vi "Save and Load Filter to and from Text File.vi"() -> ()   [LabVIEW 2023]
doc: "Demonstrates how to use the DFD Save to Text File VI to save a filter as a text file. This VI also demonstrates how to use the DFD Load from Text File VI to load a filter from a text file. \n\nComplete the following steps to use this VI.\n1) Run the VI.\n2) On the dialog box that appears, specify the path to the file in which you want to save the filter and click the <B>OK</B> button.\n3) Observe the Magnitude Responses graph. The Original Filter plot shows the magnitude response of the original filter. The Filter from File plot shows the magnitude response of the filter that the VI loads from the text file that you specified in Step 2.\n4) Examine the block diagram to learn how to use the Utilities VIs."
uses:
  <vilib>/addons/Digital Filter Design/_Objects.llb/DFD Filter Ripple Specification (Design).ctl
  <vilib>/addons/Digital Filter Design/_Objects.llb/DFD Filter Frequence Specification (Design).ctl
  <vilib>/addons/Digital Filter Design/Analysis.llb/DFD Plot Freq Response (Linear-Spaced).vi
  <vilib>/addons/Digital Filter Design/FilterLib.llb/DFD Save Filter to Text File.vi
  <vilib>/addons/Digital Filter Design/FilterLib.llb/DFD Load Filter from Text File.vi
  <vilib>/addons/Digital Filter Design/NI_DigFilterLicensed.lvlib
panel:
  out "Text":string
  in  "Load Type":u16(ring) items=["From Coefficients", "From Zero-Pole-Gain"]
  in  "Design Method":T1(ring)=enum."Elliptic"
  out "Magnitude Responses":cluster{"f0":dbl, "df":dbl, "values":dbl[]}[](graph)
  in  "Filter Type":u16(ring) items=["Lowpass", "Highpass", "Bandpass", "Bandstop"]
  in  "Frequency Sepcifications [Hz]":T2={"fpass 1"=100.0, "fstop 1"=200.0, "fpass 2 "=0.0, "fstop 2"=0.0}
  in  "Ripple Specifications":T3={"passband"=0.1, "stopband"=60.0, "dB/linear? (T: dB)"=TRUE}
  in  "Sampling Frequency [Hz]":dbl=1000.0 format="%.2f"
  out "Error Message":string
  # "Select Help>>Show Context Help and move the cursor over the VI icon for more information."
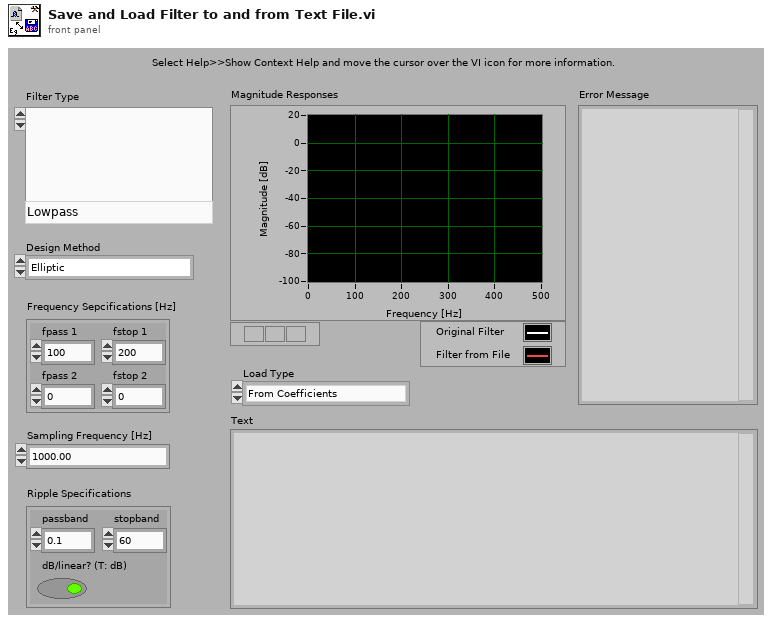
[diagram p1: front panel]
types:
  T1 = enum16{"Butterworth", "Chebyshev", "Inverse Chebyshev", "Elliptic", "Kaiser Window", "Dolph-Chebyshev Window", "Equi-Ripple FIR"}
  T2 = typedef "NI_DigFilterLicensed.lvlib/DFD Filter Frequence Specification (Design).ctl" = cluster{"fpass 1":dbl, "fstop 1":dbl, "fpass 2 ":dbl, "fstop 2":dbl}
  T3 = typedef "NI_DigFilterLicensed.lvlib/DFD Filter Ripple Specification (Design).ctl" = cluster{"passband":dbl, "stopband":dbl, "dB/linear? (T: dB)":bool}
  T4 = typedef "NI_DigFilterLicensed.lvlib/DFD Filter Obj.ctl" = cluster{"mSRate_Fs":dbl, "mSRate_Version":string, "mSRate_Comments":string, "mSRate_OrgCoef":T5, "mSRate_CurCoef":T5, "mSRate_Quantized?":bool, "mSRate_QCoef":T5, "mSRate_QSettings":T7[], "mSRate_Order":i32, "mSRate_Scaling":cluster{"mSRate_ScaleByPowerOf2?":bool, "mSRate_ScaleType":T9}}
  T5 = typedef "NI_DigFilterLicensed.lvlib/DFD Filter Coef.ctl" = cluster{"type":T6, "gain":dbl, "coef a (k)":dbl[], "coef b (v)":dbl[]}
  T6 = typedef "NI_DigFilterLicensed.lvlib/DFD Filter Structure Type Selector.ctl" = enum16{"Undefined", "FIR Direct Form", "FIR Direct Form Transposed", "FIR Symmetric", "FIR Antisymmetric", "IIR Direct Form I", "IIR Direct Form I Transposed", "IIR Direct Form II", "IIR Direct Form II Transposed", "IIR Cascaded Second Order Sections Form I", "IIR Cascaded Second Order Sections Form I Transposed", "IIR Cascaded Second Order Sections Form II", "IIR Cascaded Second Order Sections Form II Transposed", "Lattice Allpass (basic sections)", "Lattice Allpass (one multiplier sections)", "Lattice Allpass (normalized sections)", "Lattice AR (basic sections)", "Lattice AR (one multiplier sections)", "Lattice AR (normalized sections)", "Lattice MA (minimum phase)", "Lattice MA (maximum phase)", "Lattice ARMA (basic sections)", "Lattice ARMA (one multiplier sections)", "Lattice ARMA (normalized sections)"}
  T7 = typedef "NI_DigFilterLicensed.lvlib/dfd_Internal Quantization Settings.ctl" = cluster{"source":T8, "wl":i16, "iwl":i16, "overflow mode":enum16{"Saturation", "Wrap"}, "rounding mode":enum16{"Nearest", "Truncation"}, "signed?":bool}
  T8 = typedef "NI_DigFilterLicensed.lvlib/dfd_Internal Quantization Srcs.ctl" = u16
  T9 = typedef "NI_DigFilterLicensed.lvlib/DFD Coef Norm Type.ctl" = enum16{"No Norm", "Time Domain 1-Norm", "Time Domain 2-Norm", "Time Domain Inf-Norm"}
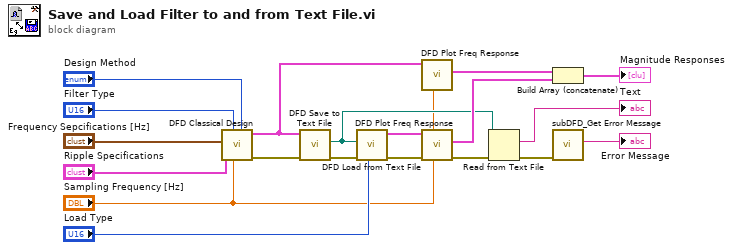
[diagram p0: block diagram]
diagram:
  n1 = call <vilib>:"DFD Classical Design.vi"("design method"="Design Method", "fs [Hz]"="Sampling Frequency [Hz]", "filter type"="Filter Type", "ripple specs"="Ripple Specifications", "freq specs [Hz]"="Frequency Sepcifications [Hz]") -> ("error out"=w11:errorcluster, "filter out"=w9:T4)  [unwired: 1 in, 4 out]
  n2 = call-poly <vilib>:"DFD Save to Text File.vi"("error in (no error)"=w11, "filter in"=w9) -> ("error out"=w12:errorcluster, "file path out"=w6:path)  [unwired: 2 in, 6 out]
  n3 = call-poly <vilib>:"DFD Load from Text File.vi"("load type"="Load Type", "error in (no error)"=w12, "file path in"=w6) -> ("error out"=w13:errorcluster, "filter out"=w14:T4)  [unwired: 7 out]
  n4 = call-poly <vilib>:"DFD Plot Freq Response.vi"("fs [Hz]"="Sampling Frequency [Hz]", "filter in"=w9) -> ("magnitude response"=w8:cluster{"f0":dbl, "df":dbl, "values":dbl[]}[])  [unwired: 6 in, 3 out]
  n5 = call-poly <vilib>:"DFD Plot Freq Response.vi"("fs [Hz]"="Sampling Frequency [Hz]", "error in (no error)"=w13, "filter in"=w14) -> ("error out"=w5:errorcluster, "magnitude response"=w7:cluster{"f0":dbl, "df":dbl, "values":dbl[]}[])  [unwired: 5 in, 2 out]
  n6 = Read from Text File(file (use dialog)=w6, error in=w5) -> (text=→"Text":string, error out=w4:errorcluster)  [unwired: 4 out]
  n7 = Build Array (concatenate)(w8, w7) -> (→"Magnitude Responses":cluster{"f0":dbl, "df":dbl, "values":dbl[]}[])
  n8 = call <vilib>:"subDFD_Get Error Message.vi"("error in (no error)"=w4) -> ("Error Message"=→"Error Message":string)  [unwired: 10 out]
